vi "Launch.vi"(10 "Actor":refnum<class "Actor.lvclass">, 11 "Panel in":refnum<class "Helper Loop.lvclass">) -> (0 "error out":errorcluster, 3 "Panel out":refnum<class "Helper Loop.lvclass">)   [LabVIEW 2021, in "Helper Loop.lvclass"]
uses:
  Helper Loop.lvclass
  <vilib>/jettl/jettl/Actor/Actor/Actor.lvclass
  Event Loop Wrapper.vi
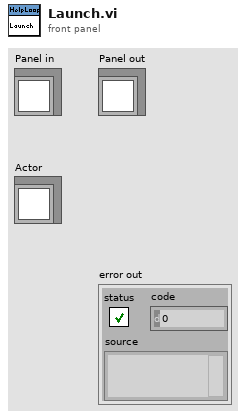
[diagram p1: front panel]
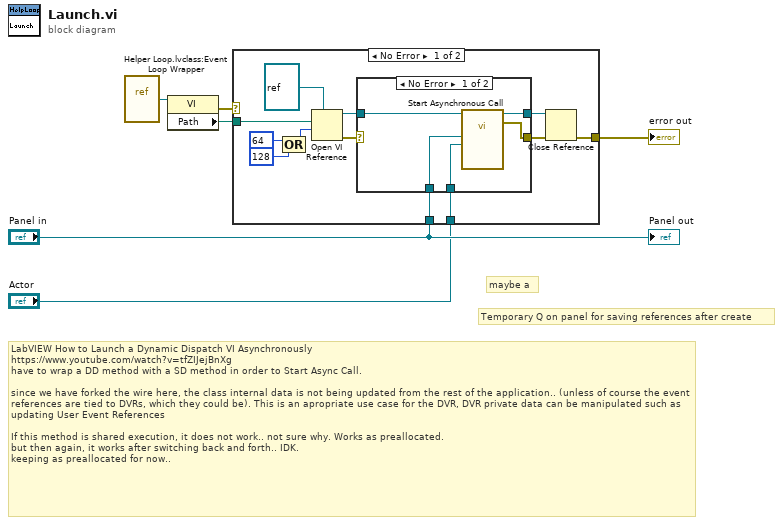
[diagram p0: block diagram]
diagram:
  # "maybe a"
  # "Temporary Q on panel for saving references after create"
  # "LabVIEW How to Launch a Dynamic Dispatch VI Asynchronously\nhttps://www.youtube.com/watch?v=tfZIJejBnXg\nhave to wrap a DD method with a SD method in order to Start Async Call.\n\nsince we have forked the wire here, the class internal data is not being updated from the rest of the application.. (unless of course the event references are tied to DVRs, which they could be). This is an apropriate use case for the DVR, DVR private data can be manipulated such as updating User Event References\n\nIf this method is shared execution, it does not work.. not sure why. Works as preallocated.\nbut then again, it works after switching back and forth.. IDK.\nkeeping as preallocated for now.."
  n1 = vi-ref "Helper Loop.lvclass:Event Loop Wrapper.vi"() -> (w2:refnum<vi>)
  n2 = property class="VI"(reference=w2) -> (error out=w3:errorcluster, "Path"=w1:path)  [unwired: 1 in, 1 out]
  n3 = case shown="No Error" w3 {
    selector: w3 -> [_ w26]
    tunnel: [w16 w26] -> w6
    tunnel: w1 -> [w9 _]
    tunnel: "Actor" -> [w8 _]
    tunnel: "Panel in" -> [w7 _]
    frame No Error {
      n4 = Compound Arithmetic op=OR(64 ("options: Multiple Clones,\n  Fire & Forget"), 128 ("options: Multiple Clones,\n  Fire & Forget")) -> (w14:i32)
      n5 = Open VI Reference(type specifier VI Refnum (for type only)=refnum<vi> refnum, vi path=w9, options=w14) -> (vi reference=w11:refnum<vi>, error out=w12:errorcluster)  [unwired: 3 in]
      n6 = case shown="No Error" w12 {
        selector: w12 -> [_ w25]
        tunnel: [w22 w24] -> w18
        tunnel: [w21 w25] -> w17
        tunnel: w11 -> [w23 w24]
        tunnel: w8 -> [w20 _]
        tunnel: w7 -> [w19 _]
        frame No Error {
          n7 = call-by-ref "Start Asynchronous Call"(reference=w23, "Actor"=w20, "Panel in"=w19) -> (reference out=w22:refnum<vi>, error out=w21:errorcluster)  [unwired: 11 in]
        }
        frame Error {
        }
      }
      n8 = Close Reference(reference=w18, error in (no error)=w17) -> (error out=w16:errorcluster)
    }
    frame Error {
    }
  }
  "error out" <- w6
  "Panel out" <- "Panel in"
